vi "Select_format_file.vi"(8 "error in (no error)":errorcluster, 10 "Formato":enum16{"TXT", "TDMS"}(ring), 11 "GUI_Actor in":refnum<class "GUI_Actor.lvclass">) -> (0 "error out":errorcluster, 3 "GUI_Actor out":refnum<class "GUI_Actor.lvclass">)   [LabVIEW 2019, in "GUI_Actor.lvlib" / "GUI_Actor.lvclass"]
uses:
  GUI_Actor.lvclass
  C:/Program Files/National Instruments/LabVIEW 2019/vi.lib/ActorFramework/Actor/Actor.lvclass
  GUI_Actor.lvclass/GUI_Actor.ctl
  Logging_txt/Logging_txt/Logging_txt.lvclass
  Logging_tdms/Logging_tdms/Logging_tdms.lvclass
  C:/Users/Luis/Documents/Ingenieria/Git_versiones/Actor-framework-CML-con-opciones-de-adquisici-n-main/Logging_txt/Logging_txt/Logging_txt.lvclass
  <vilib>/ActorFramework/Message Enqueuer/Message Enqueuer.lvclass/Message Enqueuer.ctl
  <vilib>/ActorFramework/Message Enqueuer/Enqueue.vi
  <vilib>/ActorFramework/Stop Msg/Stop Msg.lvclass
  C:/Program Files/National Instruments/LabVIEW 2019/vi.lib/ActorFramework/Message/Message.lvclass
  <vilib>/ActorFramework/Message Priority Queue/Priority Enqueue.vi
  <vilib>/ActorFramework/Actor/Actor.lvclass
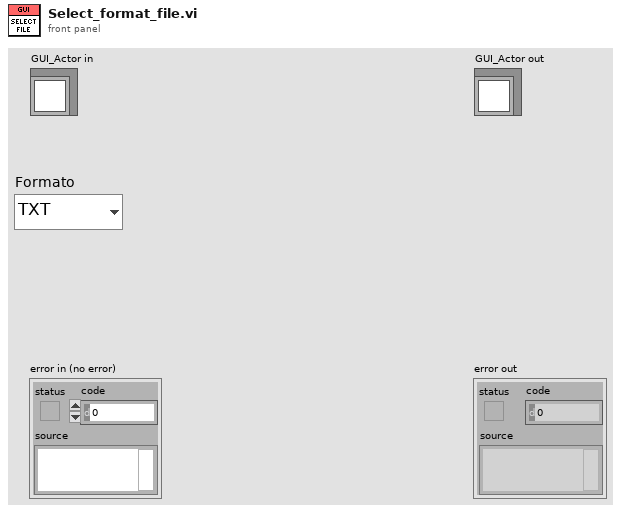
[diagram p1: front panel]
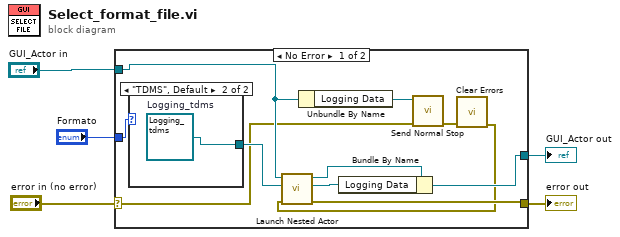
[diagram p0: block diagram]
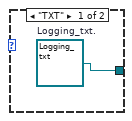
[diagram p2: hidden frame]
diagram:
  n1 = case shown="No Error" "error in (no error)" {
    selector: "error in (no error)" -> [w6 w20]
    tunnel: [w13 w20] -> w4
    tunnel: [w12 w19] -> w2
    tunnel: "GUI_Actor in" -> [w10 w19]
    tunnel: "Formato" -> [w16 _]
    frame No Error {
      n2 = case shown="\"TDMS\", Default" w16 {
        tunnel: [w17 w18] -> w14
        frame "TXT" {
          w17 = refnum<class "Logging_txt.lvclass"> refnum  # Logging_txt.
        }
        frame "TDMS", Default {
          w18 = refnum<class "Logging_tdms.lvclass"> refnum  # Logging_tdms
        }
      }
      n3 = Unbundle By Name(w10) -> ("Logging Data"=w9:refnum<class "Message Enqueuer.lvclass">)
      n4 = call <vilib>:"Send Normal Stop.vi"("error in (no error)"=w6, "Message Enqueuer"=w9) -> ("error out"=w8:errorcluster)  [unwired: 9 in]
      n5 = call <vilib>:"Clear Errors.vi"("error in (no error)"=w8) -> ("error out"=w7:errorcluster)  [unwired: 5 in, 1 out]
      n6 = call <vilib>:"Launch Nested Actor.vi"("error in (no error)"=w7, "Nested Actor"=w14, "Caller Actor in"=w10) -> ("error out"=w13:errorcluster, "Nested Actor's Enqueuer"=w11:refnum<class "Message Enqueuer.lvclass">, "Caller Actor out"=w15:refnum<class "GUI_Actor.lvclass">)  [unwired: 6 in]
      n7 = Bundle By Name(cluster=w15, "Logging Data"=w11) -> (w12:refnum<class "GUI_Actor.lvclass">)
    }
    frame Error {
    }
  }
  "error out" <- w4
  "GUI_Actor out" <- w2
